vi "2D_Flip_UD.vi"(8 "Error In":errorcluster, 11 "Array In":u16[][](array[numeric])) -> (0 "Error Out":errorcluster, 3 "Array Out":u16[][](array[numeric]))   [LabVIEW 2019]
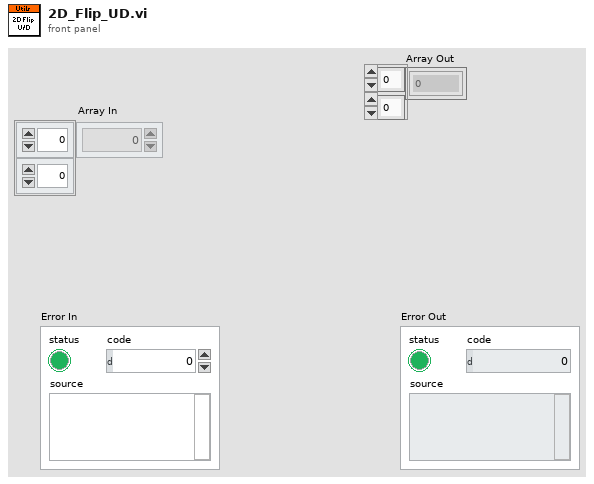
[diagram p1: front panel]
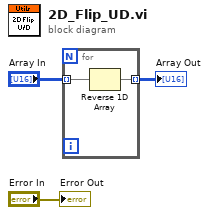
[diagram p0: block diagram]
diagram:
  n1 = for {
    tunnel: "Array In" -> [w5] mode=indexing
    tunnel: [w4] -> w2 mode=indexing
    n2 = Reverse 1D Array(array=w5) -> (reversed array=w4:u16[])
  }
  "Array Out" <- w2
  "Error Out" <- "Error In"
